vi "Icons.vi"() -> (4 "Selected":i32=37, 6 "Non Selected":i32=37)   [LabVIEW 2021, in "Measurement Builder.lvlib"]
uses:
  Measurement Builder.lvlib
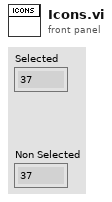
[diagram p1: front panel]
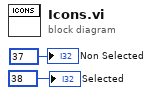
[diagram p0: block diagram]
diagram:
  "Non Selected" <- 37
  "Selected" <- 38
